vi "Add Worker VI Ref MHLC.vi"(8 "error in (no error)":errorcluster, 10 "Data in":variant, 11 "AppMgr in":refnum<class "Application Manager.lvclass">) -> (0 "error out":errorcluster, 3 "AppMgr out":refnum<class "Application Manager.lvclass">)   [LabVIEW 2017, in "Application Manager.lvclass"]
doc: "Update Worker in tree with data about Worker"
uses:
  Application Manager.lvclass
  C:/Program Files (x86)/National Instruments/LabVIEW 2017/vi.lib/addons/_Workers/Library/Classes/Worker/Worker.lvclass
  <vilib>/addons/_Workers/Library/Classes/Worker/Worker Debug Data.ctl
  <vilib>/addons/_Workers/Library/Classes/Worker/Worker Type.ctl
  <vilib>/addons/_Workers/Library/Classes/Message Queue/Message Queue.lvclass
  <vilib>/addons/_Workers/Library/Classes/Worker/Worker Status.ctl
  <vilib>/addons/_Workers/Library/Classes/Worker/Worker.lvclass/Worker.ctl
  <vilib>/addons/_Workers/Library/Classes/Message/Message.lvclass/Message.ctl
  Application Manager.lvclass/Application Manager.ctl
  <vilib>/addons/_Workers/Library/Classes/Worker/Read Message.vi
  <vilib>/addons/_Workers/Library/Classes/Message/Read Sender WID.vi
  Common VIs/DC Name to DC_UID.vi
  <vilib>/Utility/error.llb/Error Cluster From Error Code.vi
  <vilib>/ErrorRing/Error Ring.xnode
  <vilib>/addons/_Workers/Library/Classes/Worker/Worker.lvclass
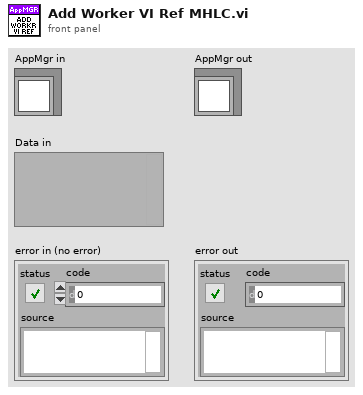
[diagram p1: front panel]
types:
  T1 = typedef "Workers.lvlib/Worker.lvclass/Worker Status.ctl" = enum16{"Queue created", "Preinitialized", "Initialize called", "Initialized", "Start Exiting called", "Exited", "Stopped (Critical Error)"}
  T2 = typedef "Workers.lvlib/Worker.lvclass/Worker Debug Data.ctl" = cluster{"WID":string, "VI Ref":refnum<vi>, "VI Path":path, "CloneID":string, "Type":T3, "Queue":refnum<class "Message Queue.lvclass">}
  T3 = typedef "Workers.lvlib/Worker.lvclass/Worker Type.ctl" = enum16{"SL", "DL"}
  T4 = typedef "Application Manager.lvclass/Debug Client Data.ctl" = cluster{"DC_UID":T5, "IP Address":string, "Worker Data":T6[], "Connected":bool}
  T5 = typedef "DC_UID.ctl" = string
  T6 = typedef "Application Manager.lvclass/Worker Data.ctl" = cluster{"ID":string, "VI Ref":refnum<vi>, "VI Path":path, "CloneID":string, "Type":T3, "Worker Status":string}
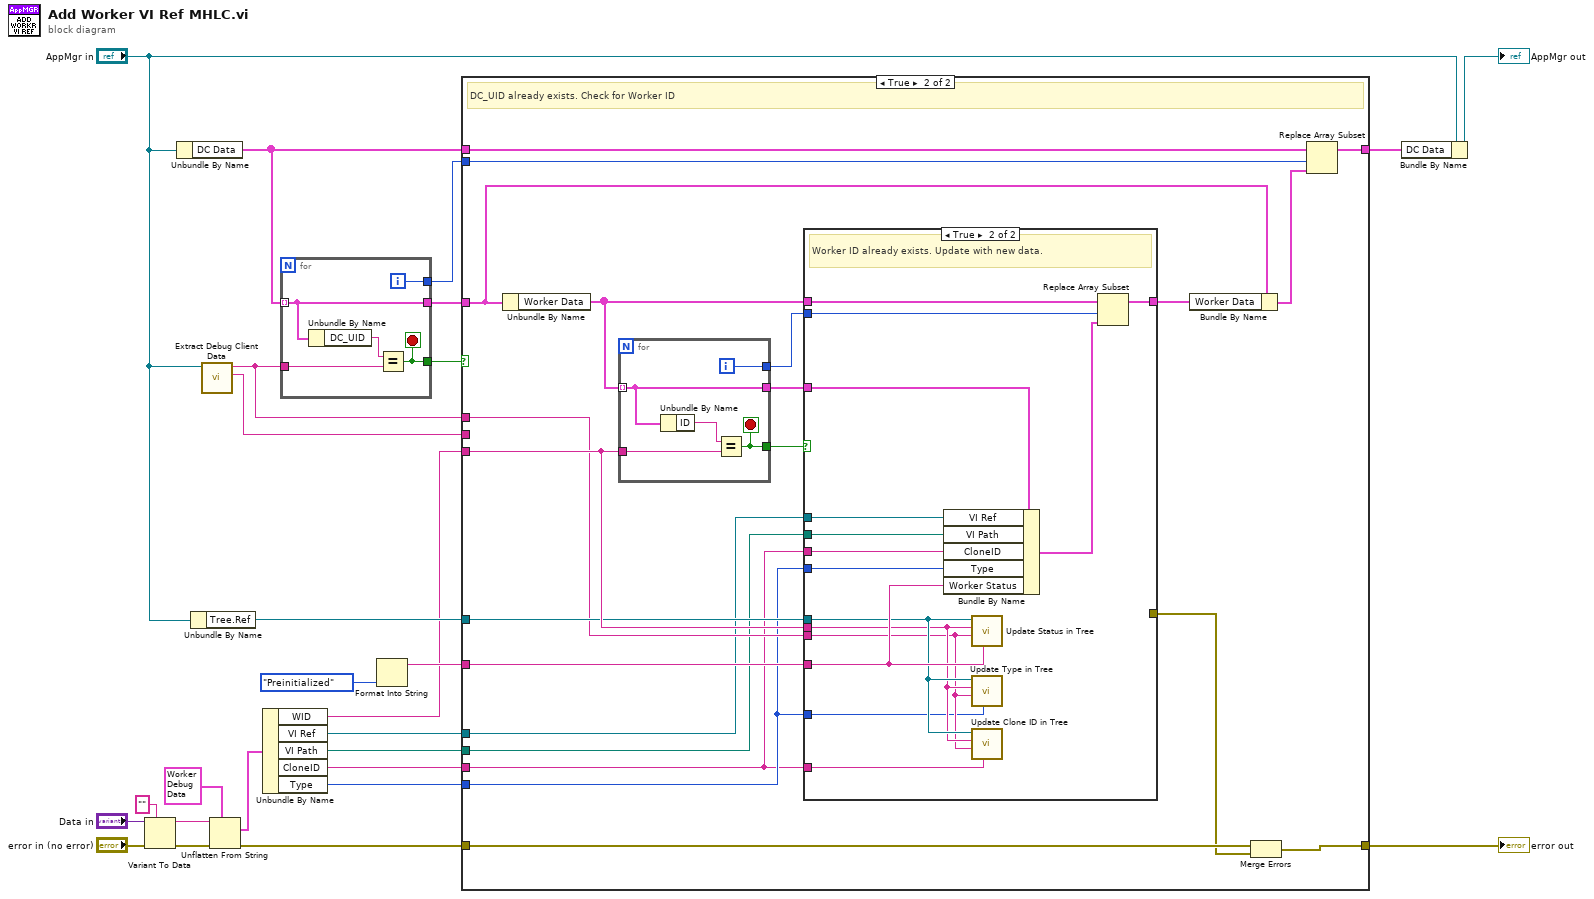
[diagram p0: block diagram]
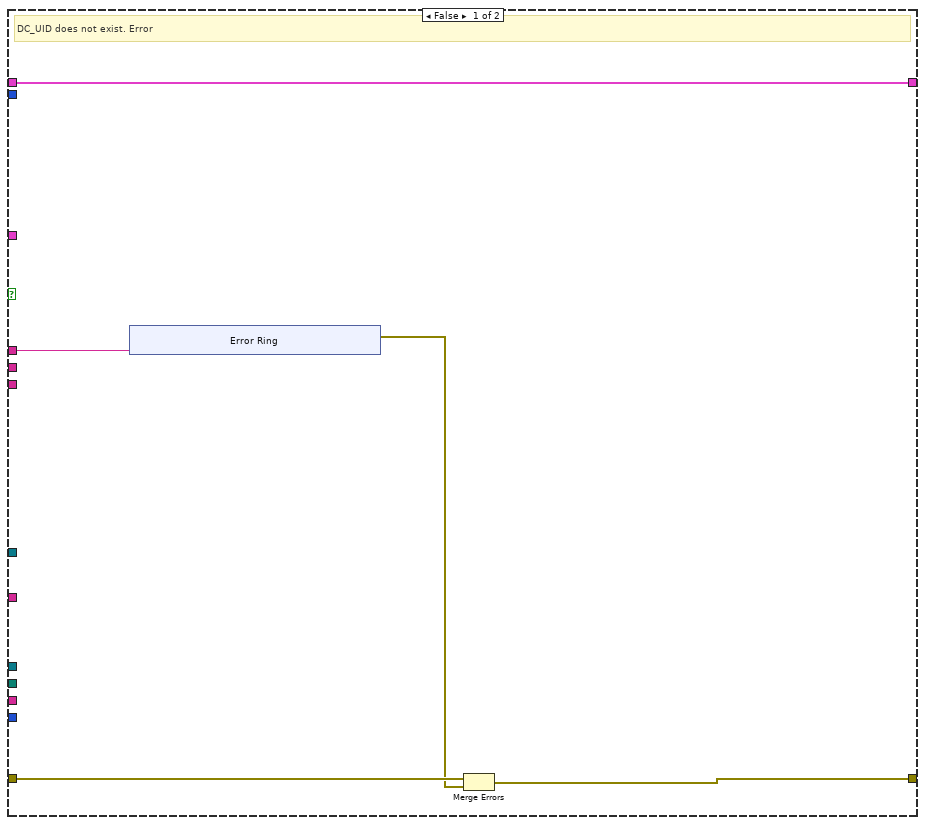
[diagram p2: hidden frame]
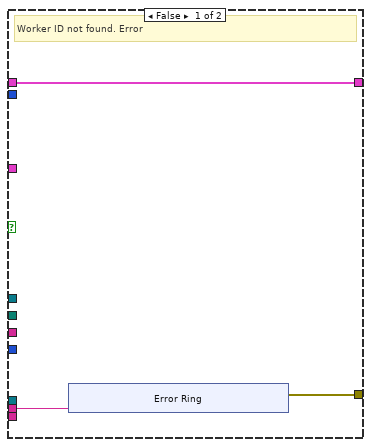
[diagram p3: hidden frame]
diagram:
  n1 = Variant To Data(error in="error in (no error)", type="", Variant="Data in") -> (data=w22:string, error out=w23:errorcluster)
  n2 = Unbundle By Name("AppMgr in") -> ("DC Data"=w20:T4[])
  n3 = Unbundle By Name("AppMgr in") -> ("Tree.Ref"=w17:refnum<vi>)
  n4 = call "Extract Debug Client Data.vi"("AppMgr in"="AppMgr in") -> ("IP Address"=w18:string, "DC_UID"=w19:T5)  [unwired: 9 in]
  n5 = Unflatten From String(type=T2 {"WID"="", "VI Ref"=refnum, "VI Path"=path "", "CloneID"="", "Type"=enum."SL", "Queue"=refnum} ("Worker VI Ref Data"), binary string=w22, error in (no error)=w23) -> (value=w8:T2, error out=w5:errorcluster)  [unwired: 2 in, 1 out]
  n6 = Unbundle By Name(w8) -> ("WID"=w7:string, "VI Ref"=w4:refnum<vi>, "VI Path"=w3:path, "CloneID"=w2:string, "Type"=w1:T3)
  n7 = for {
    tunnel: w20 -> [w27] mode=indexing
    tunnel: w19 -> [w30]
    tunnel: [w29] -> w11
    tunnel: [w28] -> w16
    tunnel: [w27] -> w14
    i -> [w28]
    stop <- w29 stop-if-true
    n8 = Unbundle By Name(w27) -> ("DC_UID"=w31:T5)
    n9 = Equal?(x=w31, y=w30) -> (x = y?=w29:bool)
  }
  n10 = Format Into String(Worker_Status."Preinitialized" ("Worker Status")) -> (resulting string=w12:string)  [unwired: 3 in, 1 out]
  n11 = case shown="True" w11 {
    tunnel: w20 -> [w36 w64]
    tunnel: w19 -> [w32 w51]
    tunnel: w7 -> [_ w55]
    tunnel: w18 -> [_ _]
    tunnel: w17 -> [_ w52]
    tunnel: w16 -> [_ w62]
    tunnel: [w36 w63] -> w15
    tunnel: w14 -> [_ w60]
    tunnel: w12 -> [_ w54]
    tunnel: [w34 w49] -> w6
    tunnel: w5 -> [w35 w50]
    tunnel: w4 -> [_ w47]
    tunnel: w3 -> [_ w46]
    tunnel: w2 -> [_ w44]
    tunnel: w1 -> [_ w45]
    frame False {
      # "DC_UID does not exist. Error"
      n12 = xnode "Error Ring"("parameter 0"=w32) -> ("error out"=w33:errorcluster)
      n13 = Merge Errors(w35, w33) -> (w34:errorcluster)
    }
    frame True {
      # "DC_UID already exists. Check for Worker ID"
      n14 = Unbundle By Name(w60) -> ("Worker Data"=w58:T6[])
      n15 = for {
        tunnel: w58 -> [w90] mode=indexing
        tunnel: w55 -> [w93]
        tunnel: [w92] -> w61
        tunnel: [w91] -> w56
        tunnel: [w90] -> w53
        i -> [w91]
        stop <- w92 stop-if-true
        n16 = Unbundle By Name(w90) -> ("ID"=w94:string)
        n17 = Equal?(x=w94, y=w93) -> (x = y?=w92:bool)
      }
      n18 = case shown="True" w61 {
        tunnel: w58 -> [w67 w89]
        tunnel: [w67 w88] -> w57
        tunnel: w56 -> [_ w87]
        tunnel: w55 -> [w66 w78]
        tunnel: w54 -> [_ w84]
        tunnel: w53 -> [_ w86]
        tunnel: w52 -> [_ w79]
        tunnel: w51 -> [_ w77]
        tunnel: [w65 _] -> w48
        tunnel: w47 -> [_ w83]
        tunnel: w46 -> [_ w82]
        tunnel: w44 -> [_ w81]
        tunnel: w45 -> [_ w80]
        tunnel: w45 -> [_ w76]
        tunnel: w44 -> [_ w75]
        frame False {
          # "Worker ID not found. Error"
          n19 = xnode "Error Ring"("parameter 0"=w66) -> ("error out"=w65:errorcluster)
        }
        frame True {
          # "Worker ID already exists. Update with new data."
          n20 = Bundle By Name(cluster=w86, "VI Ref"=w83, "VI Path"=w82, "CloneID"=w81, "Type"=w80, "Worker Status"=w84) -> (w85:T6)
          n21 = call "Update Status in Tree.vi"("Worker Status"=w84, "DC_UID"=w77, "WID"=w78, "Tree Ref"=w79) -> ()  [unwired: 7 in, 1 out]
          n22 = call "Update Type in Tree.vi"("Type"=w76, "DC_UID"=w77, "WID"=w78, "Tree Ref"=w79) -> ()  [unwired: 7 in, 1 out]
          n23 = call "Update Clone ID in Tree.vi"("Clone ID"=w75, "DC_UID"=w77, "WID"=w78, "Tree Ref"=w79) -> ()  [unwired: 7 in, 1 out]
          n24 = Replace Array Subset(array=w89, new element=w85, index=w87) -> (w88:T6[])
        }
      }
      n25 = Bundle By Name(cluster=w60, "Worker Data"=w57) -> (w59:T4)
      n26 = Merge Errors(w50, w48) -> (w49:errorcluster)
      n27 = Replace Array Subset(array=w64, new element=w59, index=w62) -> (w63:T4[])
    }
  }
  "error out" <- w6
  n28 = Bundle By Name(cluster="AppMgr in", "DC Data"=w15) -> (→"AppMgr out":refnum<class "Application Manager.lvclass">)
